vi "Image Denoising.vi"() -> ()   [LabVIEW 2023]
doc: "This example shows how to reduce noise of an image with the WA Denoise VI. The flower image is contaminated by some Gaussian white noise with a standard deviation 5. This example uses the undecimated wavelet transform-based method to denoise the image.\n\n<b>Instructions:</b>\n1) Run this VI.\n2) Compare the noisy image and denoised image with different settings."
uses:
  Images/_Images.ctl
  <vilib>/addons/Wavelet Analysis/application.llb/WA Denoise (UWT 2D Array).vi
  <vilib>/addons/_Advanced Signal Processing/NI_AdvSigProcWA.lvlib
  <vilib>/vision/NI_Vision_Development_Module.lvlib
panel:
  out "output cluster 2":T1
  out "output cluster":T1
  out "Image 5":T2(plugin-control)
  out "Image 4":T2(plugin-control)
  out "Image 3":T2(plugin-control)
  out "Image 3":T2(plugin-control)
  out "Image 2":T2(plugin-control)
  out "Image":T2(plugin-control)
  in  "Threshold settings":T3={"Thresholding Rule"=enum."SURE", "Rescaling Method"=enum."Single level", "Soft Threshold?"=TRUE}
  in  "Wavelet":u16(ring) items=["db02"=0, "db03"=1, "db04"=2, "db05"=3, "db06"=4, "db07"=5, "db08"=6, "db09"=7, "db10"=8, "db11"=9, "db12"=10, "db13"=11, "db14"=12, "Haar"=13, "bior1_3"=14, "bior1_5"=15, "bior2_2"=16, "bior2_4"=17, "bior2_6"=18, "bior2_8"=19, "bior3_1"=20, "bior3_3"=21, "bior3_5"=22, "bior3_7"=23, "bior3_9"=24, "bior4_4 (FBI)"=25, "bior5_5"=38, "bior6_8"=39, "coif1"=26, "coif2"=27, "coif3"=28, "coif4"=29, "coif5"=30, "sym2"=31, "sym3"=32, "sym4"=33, "sym5"=34, "sym6"=35, "sym7"=36, "sym8"=37]
  in  "Levels":i32=4
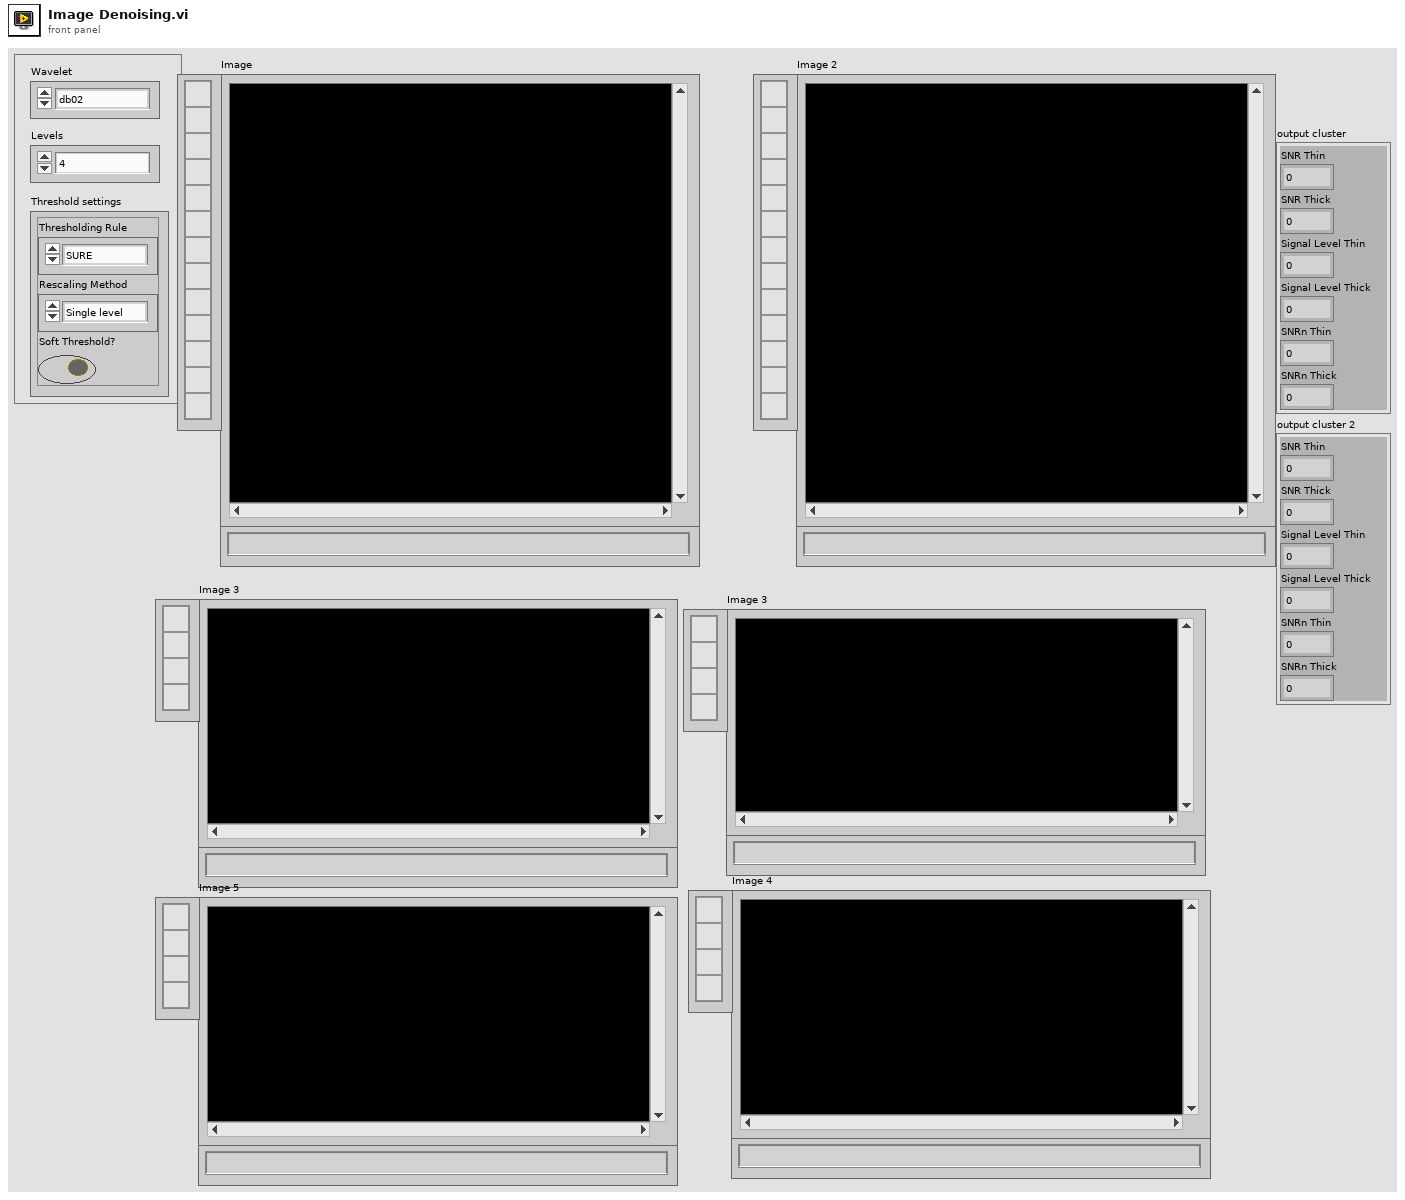
[diagram p1: front panel]
types:
  T1 = cluster{"SNR Thin":sgl, "SNR Thick":sgl, "Signal Level Thin":sgl, "Signal Level Thick":sgl, "SNRn Thin":sgl, "SNRn Thick":sgl}
  T2 = typedef "IMAQ Image.ctl" = refnum<image>
  T3 = cluster{"Thresholding Rule":enum16{"SURE", "Hybrid", "Universal", "Minimax"}, "Rescaling Method":enum16{"One", "Single level", "Multiple levels"}, "Soft Threshold?":bool}
  T4 = typedef "Image Type" = u32
  T5 = typedef "_Images.ctl" = enum16{"Balls2", "Battery1", "Battery2", "Connector1", "Subwoofer1", "Subwoofer2", "Subwoofer3", "Subwoofer4", "Hase1", "Lamp1", "Lamp2", "Mouse1", "PhotoLens1", "Po1", "PowerSupply1", "Router", "--- Step Wedges ---", "Stepwedge1", "Stepwedge2", "Stepwedge3", "--- Fusion ---", "Fusion160kV", "Fusion2-120kV", "Fusion2-320kV", "Fusion300kV", "FusionPart1-120kV", "FusionPart1-180kV", "--- PART 01 ---", "Part1", "Part2", "Part3", "Part4", "Part5", "Part6", "Part7", "Part8", "--- Different Integrations ---", "Step2737-02Int", "Step2737-04Int", "Step2737-08Int", "Step2737-16Int", "Step2737-32Int", "Step2737-64Int"}
  T6 = cluster{"Global Rectangle":i32[], "Contours":cluster{"Contour Type":u32, "ROI Type":u32, "Points":i32[]}[]}
  T7 = typedef "IMAQ Rectangle" = cluster{"Left":i32, "Top":i32, "Right":i32, "Bottom":i32, "Rotation":dbl}
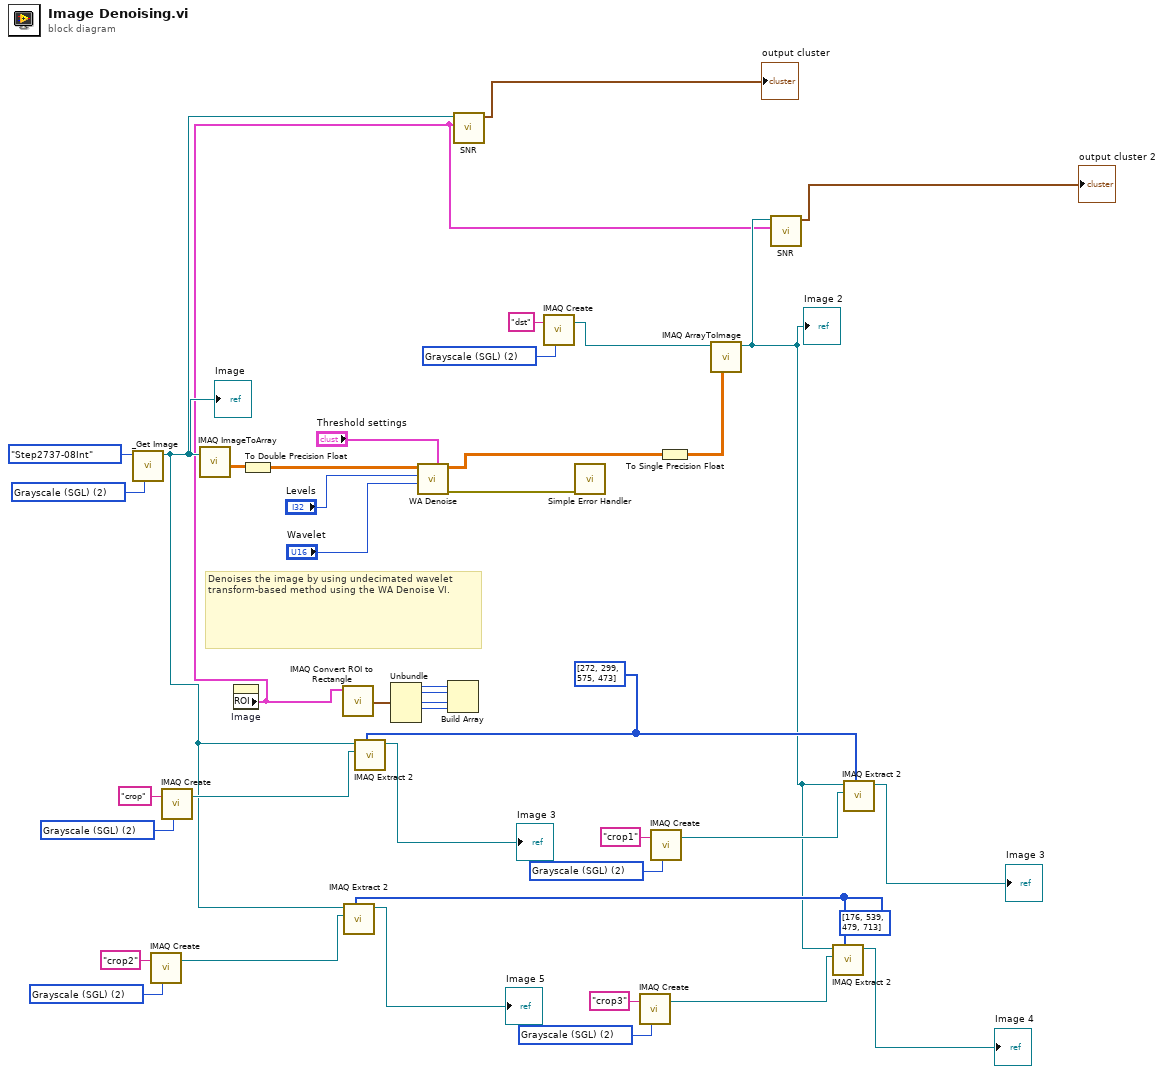
[diagram p0: block diagram]
diagram:
  w6 = i32[] [176, 539, 479, 713] ("appended array")
  w13 = T4 2 items=["Grayscale (U8)", "Grayscale (I16)", "Grayscale (SGL)", "Complex (CSG)", "RGB (U32)", "HSL (U32)", "RGB (U64)", "Grayscale (U16)"] ("Image Type")
  w7 = T4 2 items=["Grayscale (U8)", "Grayscale (I16)", "Grayscale (SGL)", "Complex (CSG)", "RGB (U32)", "HSL (U32)", "RGB (U64)", "Grayscale (U16)"] ("Image Type")
  w15 = i32[] [272, 299, 575, 473] ("appended array")
  w17 = T4 2 items=["Grayscale (U8)", "Grayscale (I16)", "Grayscale (SGL)", "Complex (CSG)", "RGB (U32)", "HSL (U32)", "RGB (U64)", "Grayscale (U16)"] ("Image Type")
  w23 = T4 2 items=["Grayscale (U8)", "Grayscale (I16)", "Grayscale (SGL)", "Complex (CSG)", "RGB (U32)", "HSL (U32)", "RGB (U64)", "Grayscale (U16)"] ("Image Type")
  w30 = T4 2 items=["Grayscale (U8)", "Grayscale (I16)", "Grayscale (SGL)", "Complex (CSG)", "RGB (U32)", "HSL (U32)", "RGB (U64)", "Grayscale (U16)"] ("Image Type")
  w35 = T4 2 items=["Grayscale (U8)", "Grayscale (I16)", "Grayscale (SGL)", "Complex (CSG)", "RGB (U32)", "HSL (U32)", "RGB (U64)", "Grayscale (U16)"] ("Image Type (U16)")
  # "Denoises the image by using undecimated wavelet transform-based method using the WA Denoise VI."
  n1 = call "_Get Image.vi"("Image Type (U16)"=w35, "Image"=_Images."Step2737-08Int") -> ("Image Out"=w5:T2)  [unwired: 6 in, 3 out]
  "Image" <- w5
  n2 = call "IMAQ Create"("Image Name"="crop2", "Image Type"=w7) -> ("New Image"=w9:T2)  [unwired: 3 in, 1 out]
  n3 = call "IMAQ Create"("Image Name"="crop", "Image Type"=w23) -> ("New Image"=w21:T2)  [unwired: 3 in, 1 out]
  n4 = call "IMAQ ImageToArray"("Image"=w5) -> ("Image Pixels (Float)"=w34:sgl[][])  [unwired: 3 in, 4 out]
  n5 = property on="Image" class="ImageControl"() -> ("ROI"=w1:T6)  [unwired: 2 in, 2 out]
  n6 = To Double Precision Float(number=w34) -> (double precision float=w37:dbl[][])
  n7 = call "IMAQ Convert ROI to Rectangle"("ROI Descriptor"=w1) -> ("Rectangle"=w28:T7)  [unwired: 8 in, 1 out]
  n8 = call "IMAQ Extract 2"("Optional Rectangle"=w6, "Image Dst"=w9, "Image Src"=w5) -> ("Image Dst Out"=→"Image 5":T2)  [unwired: 7 in, 1 out]
  n9 = call "IMAQ Extract 2"("Optional Rectangle"=w15, "Image Dst"=w21, "Image Src"=w5) -> ("Image Dst Out"=→"Image 3":T2)  [unwired: 7 in, 1 out]
  n10 = Unbundle(w28) -> ("Left"=w27:i32, "Top"=w26:i32, "Right"=w25:i32, "Bottom"=w24:i32)  [unwired: 1 out]
  n11 = call-poly <vilib>:"WA Denoise.vi"("threshold settings"="Threshold settings", "wavelet"="Wavelet", "levels"="Levels", "signal"=w37) -> ("error out"=w38:errorcluster, "denoised signal"=w32:dbl[][])  [unwired: 1 in, 5 out]
  n12 = Build Array(w27, w26, w25, w24) -> ()  [unwired: 1 out]
  n13 = call "SNR.vi"("ROI"=w1, "Refnum in"=w5) -> ("SNR Results"=→"output cluster":T1)  [unwired: 9 in]
  n14 = call "IMAQ Create"("Image Name"="dst", "Image Type"=w30) -> ("New Image"=w31:T2)  [unwired: 3 in, 1 out]
  n15 = call <vilib>:"Simple Error Handler.vi"("error in (no error)"=w38) -> ()  [unwired: 4 in, 5 out]
  n16 = call "IMAQ Create"("Image Name"="crop3", "Image Type"=w13) -> ("New Image"=w11:T2)  [unwired: 3 in, 1 out]
  n17 = call "IMAQ Create"("Image Name"="crop1", "Image Type"=w17) -> ("New Image"=w19:T2)  [unwired: 3 in, 1 out]
  n18 = To Single Precision Float(number=w32) -> (single precision float=w29:sgl[][])
  n19 = call "IMAQ ArrayToImage"("Image Pixels (Float)"=w29, "Image"=w31) -> ("Image Out"=w2:T2)  [unwired: 8 in, 1 out]
  "Image 2" <- w2
  n20 = call "SNR.vi"("ROI"=w1, "Refnum in"=w2) -> ("SNR Results"=→"output cluster 2":T1)  [unwired: 9 in]
  n21 = call "IMAQ Extract 2"("Optional Rectangle"=w6, "Image Dst"=w11, "Image Src"=w2) -> ("Image Dst Out"=→"Image 4":T2)  [unwired: 7 in, 1 out]
  n22 = call "IMAQ Extract 2"("Optional Rectangle"=w15, "Image Dst"=w19, "Image Src"=w2) -> ("Image Dst Out"=→"Image 3":T2)  [unwired: 7 in, 1 out]
